vi "ContextHelp_PopUp.vi"() -> ()   [LabVIEW 2012]
uses:
  <resource>/Framework/Providers/Open_GDS/UML/ContextHelp/ContextHelp_EventType.ctl
  <resource>/Framework/Providers/Open_GDS/UML/ContextHelp/ContextHelp_ShowType.ctl
  <vilib>/event_ctls.llb/eventvkey.ctl
panel:
  in  "CallerRef":refnum<vi>
  in  "OccSync":refnum<k4>
  in  "Event":T1
  out "new picture":picture
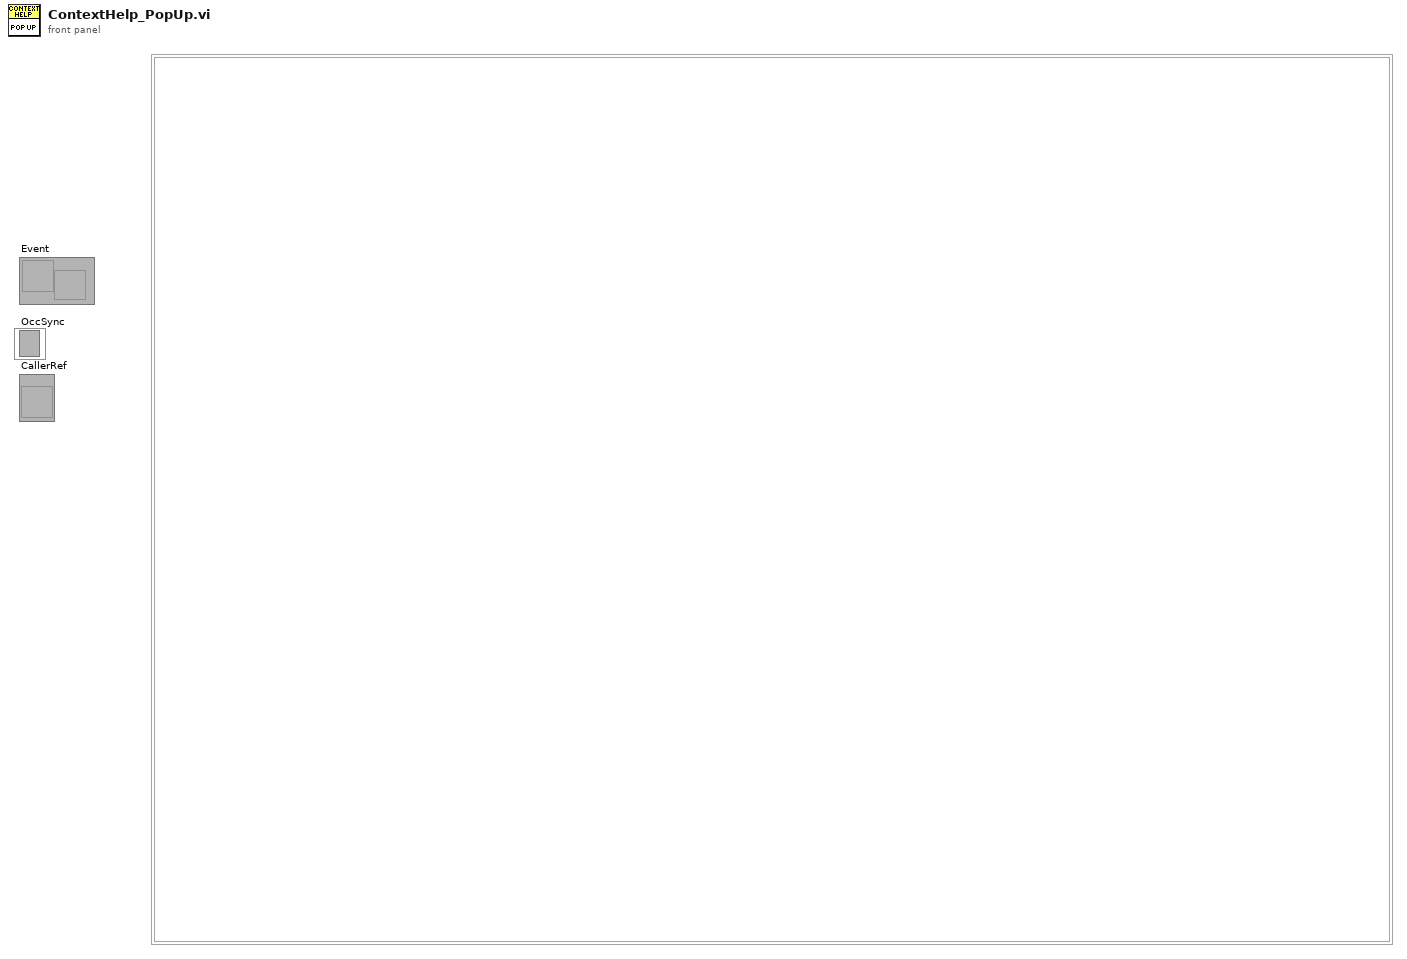
[diagram p1: front panel]
types:
  T1 = typedef "ContextHelp_EventType.ctl" = refnum<user-event>
  T2 = typedef "ContextHelp_ShowType.ctl" = cluster{"Header":string, "Picture":picture, "Text":string}
  T3 = cluster{"VIs":refnum<vi>[], "ViPathes":path[], "VI":i32, "Show":T2, "Win":cluster{"left":i16, "top":i16, "right":i16, "bottom":i16}, "LastViRef":refnum<vi>}
  T4 = enum32{"Custom", "Standard", "Using Panel", "Using SubVI", "Complete"}
  T5 = enum16{"SetPopUpEventTask", "GetStatus", "SetOpenState"}
  T6 = cluster{"left":i16, "top":i16, "right":i16, "bottom":i16}
  T7 = typedef "eventvkey.ctl" = enum16{"ASCII", "Enter", "Return", "Shift", "Ctrl", "Alt", "Cmd", "Opt", "Caps", "NumLock", "Clear", "Break", "Up", "Down", "Left", "Right", "Insert", "Delete", "Home", "End", "PageUp", "PageDown", "Escape", "Help", "Pause", "ScrollLock", "F1", "F2", "F3", "F4", "F5", "F6", "F7", "F8", "F9", "F10", "F11", "F12", "F13", "F14", "F15", "F16", "F17", "F18", "F19", "F20", "F21", "F22", "F23", "F24", "Play", "VolumeUp", "VolumeDown", "Mute", "Two Byte Char"}
  T8 = typedef "Librarian File Info Out.ctl" = cluster{"creation date":u32, "last mod date":u32, "type":string, "creator":string, "LV version":i32, "size":i32, "top level":bool}
  T9 = typedef "imagedata.ctl" = cluster{"image type":i32, "image depth":i32, "image":u8[], "mask":u8[], "colors":u32[], "Rectangle":cluster{"left":i16, "top":i16, "right":i16, "bottom":i16}}
  T10 = cluster{"Font Name:":string, "Size":i16, "Strikeout?":bool, "Italic?":bool, "Underline?":bool, "Outline?":bool, "Shadow?":bool, "Bold?":bool}
  T11 = enum16{"User-specified Font", "Application Font", "System Font", "Dialog Font"}
  T12 = typedef "LVRectTypeDef.ctl" = cluster{"Left":i16, "Top":i16, "Right":i16, "Bottom":i16}
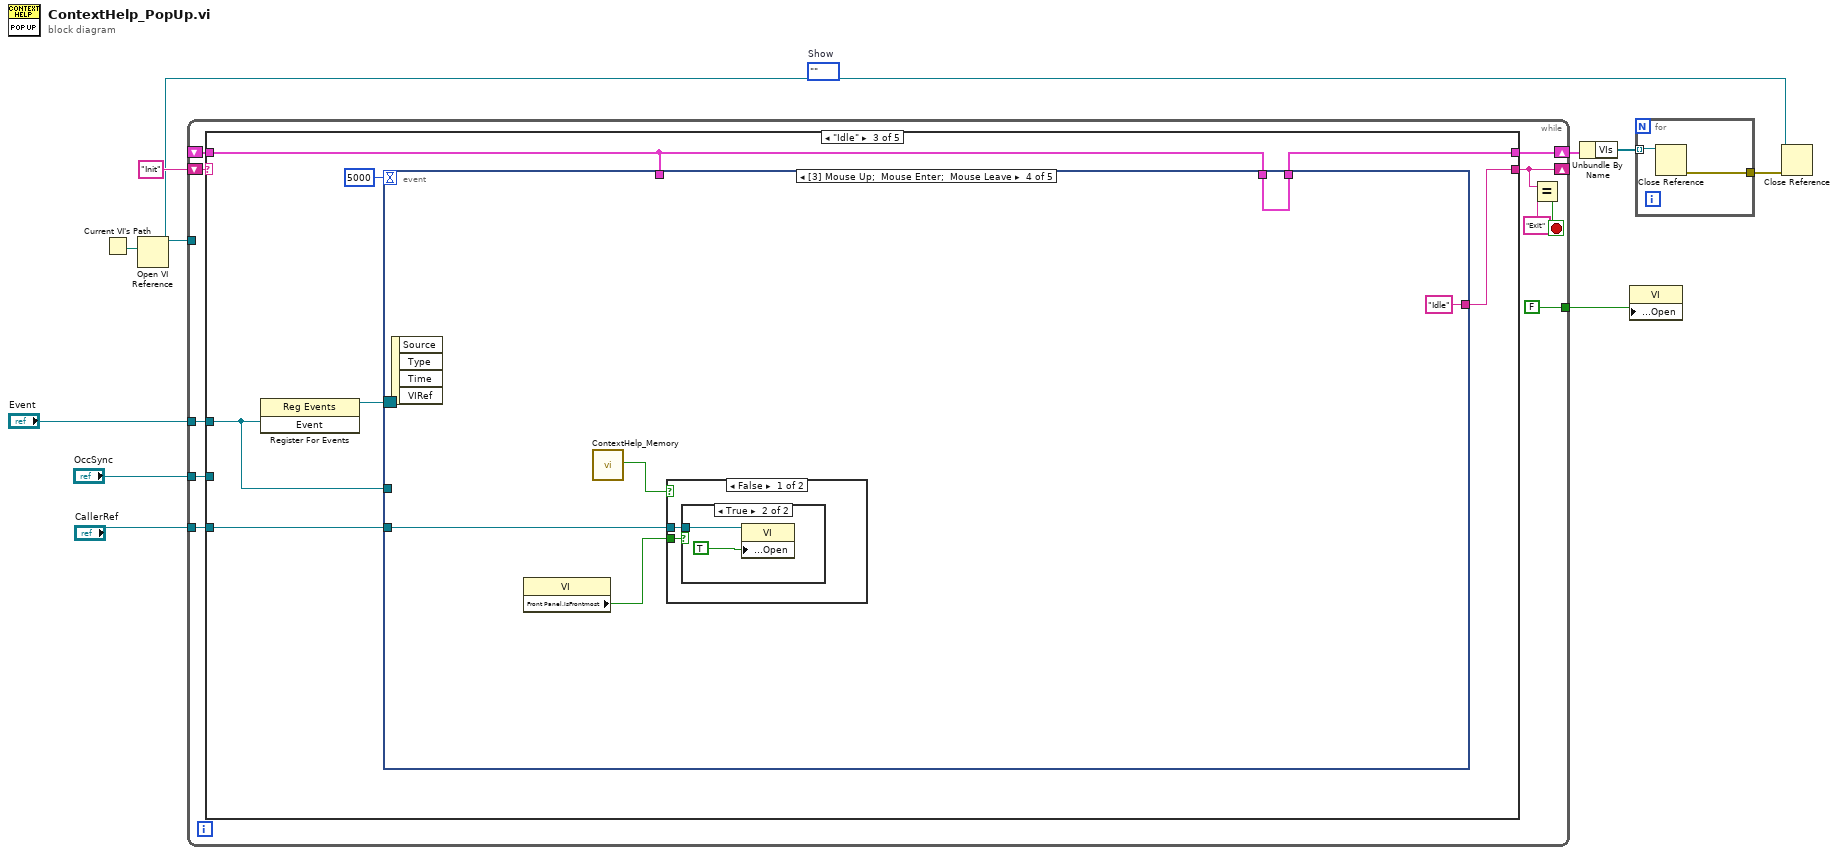
[diagram p0: block diagram]
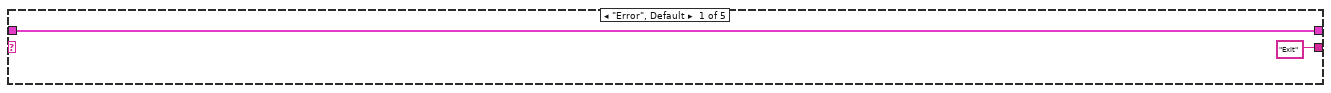
[diagram p2: hidden frame]
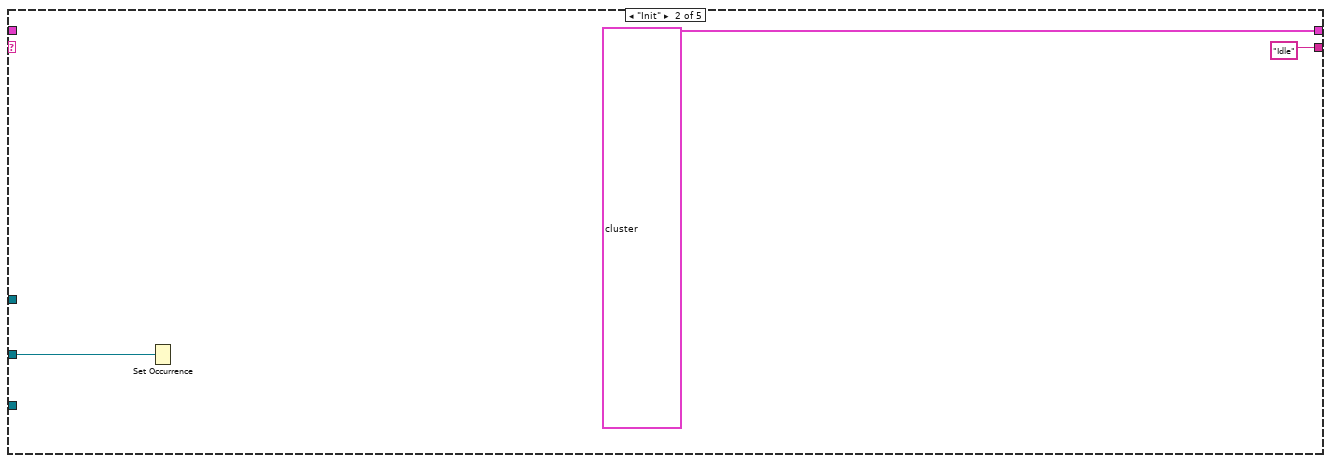
[diagram p3: hidden frame]
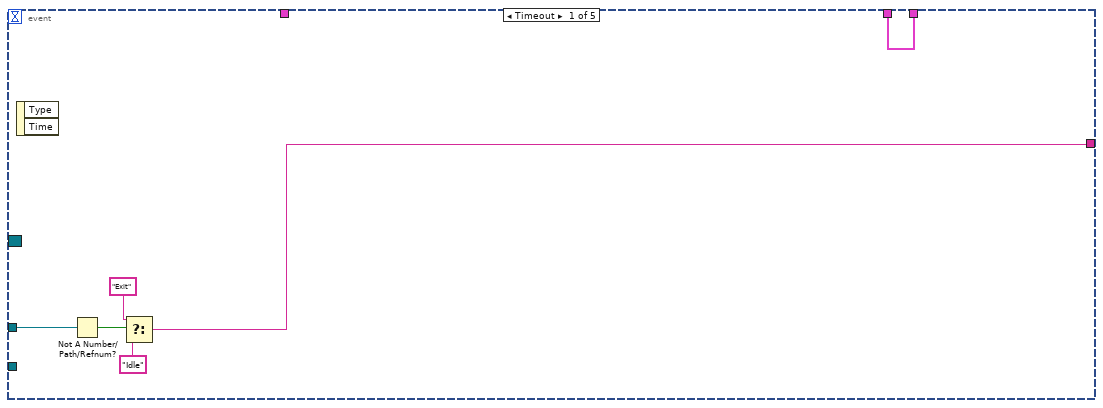
[diagram p4: hidden frame]
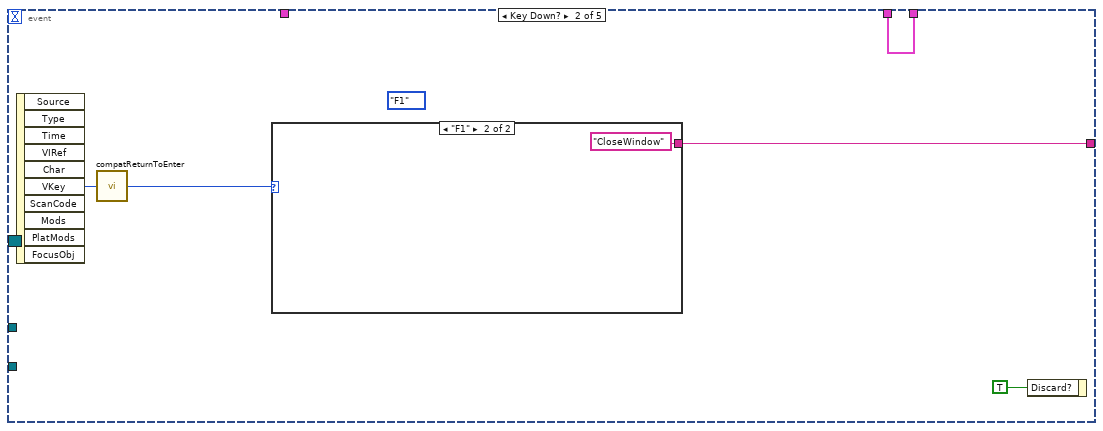
[diagram p5: hidden frame]
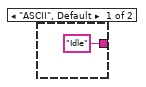
[diagram p6: hidden frame]
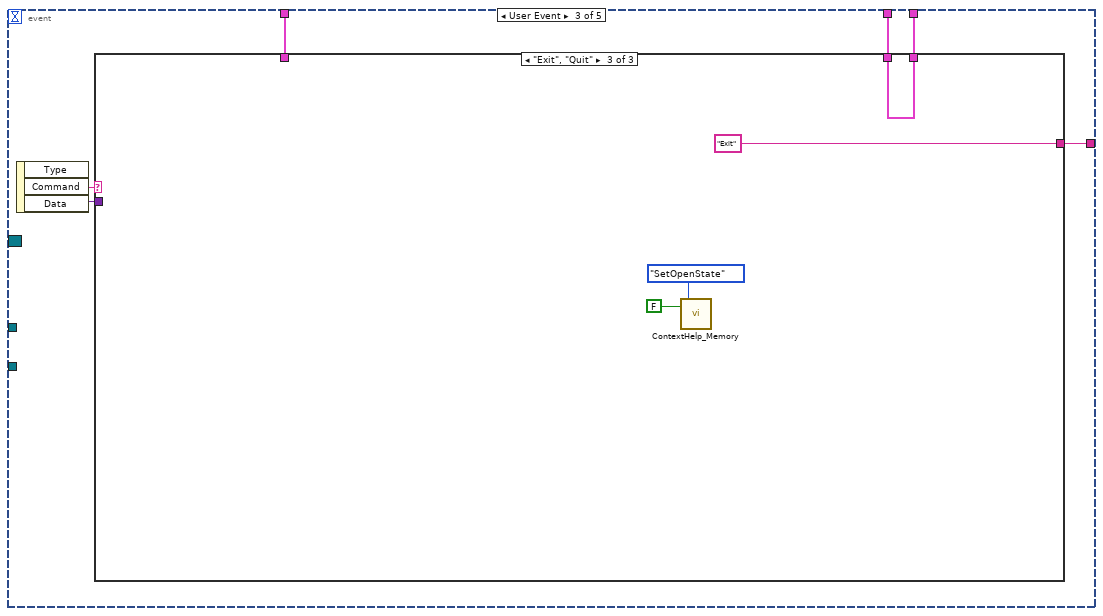
[diagram p7: hidden frame]
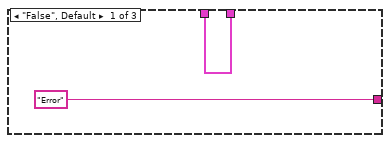
[diagram p8: hidden frame]
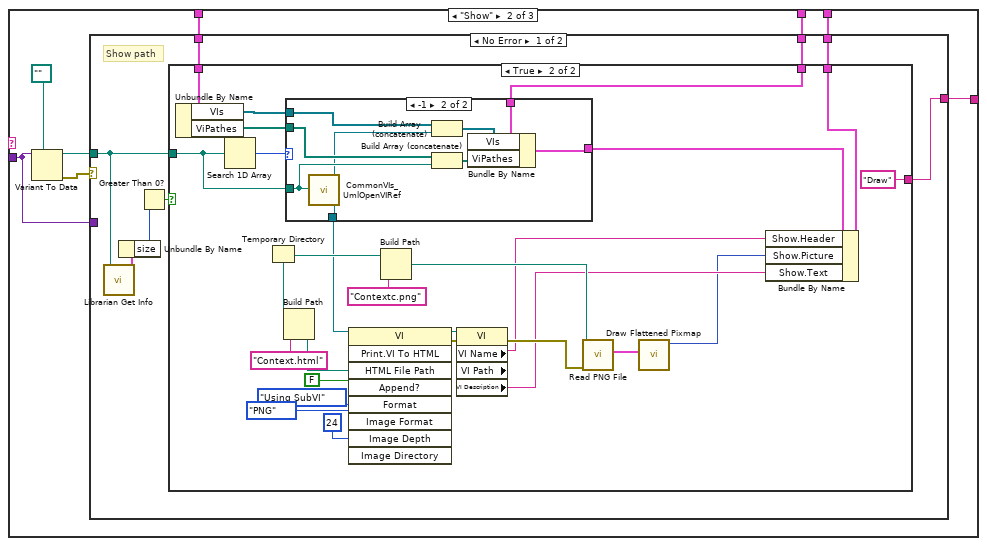
[diagram p9: hidden frame]
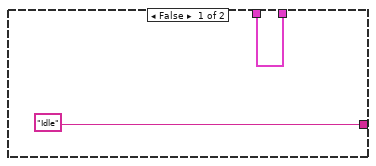
[diagram p10: hidden frame]
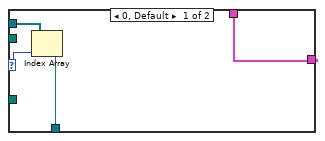
[diagram p11: hidden frame]
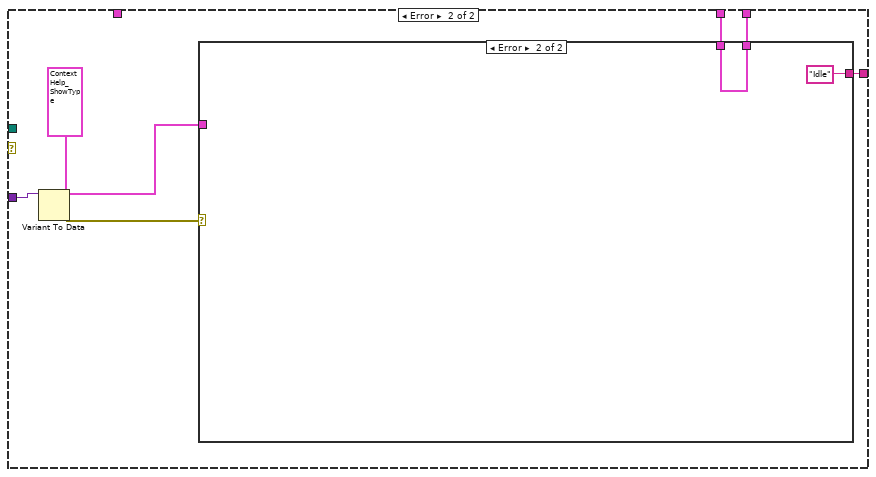
[diagram p12: hidden frame]
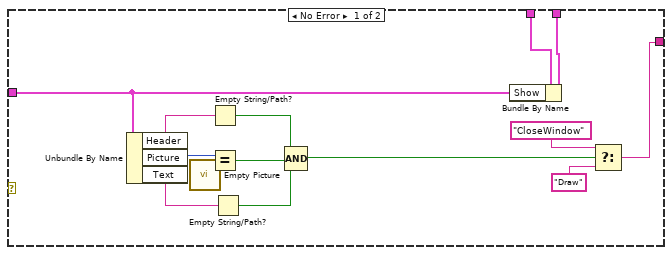
[diagram p13: hidden frame]
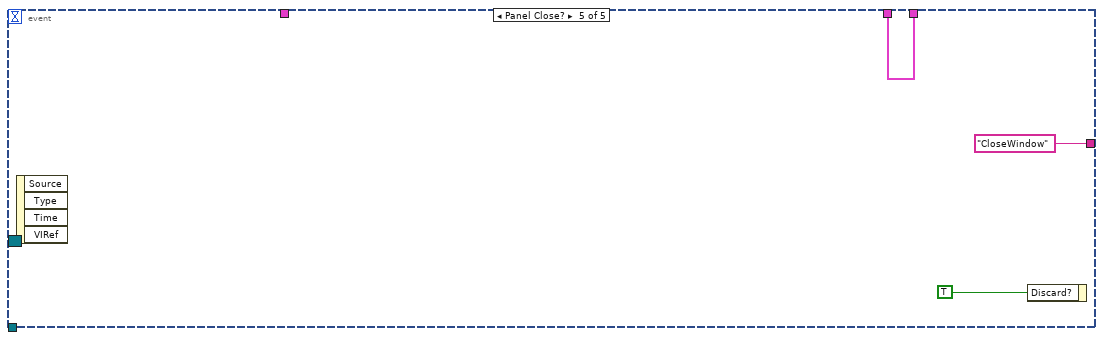
[diagram p16: hidden frame]
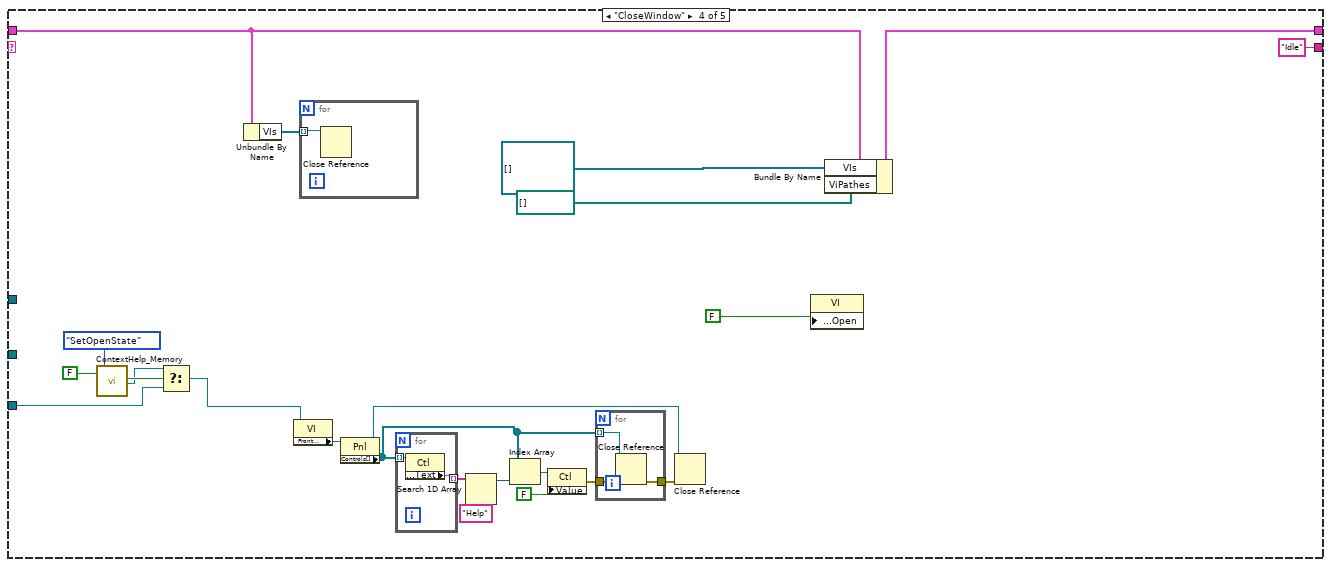
[diagram p17: hidden frame]
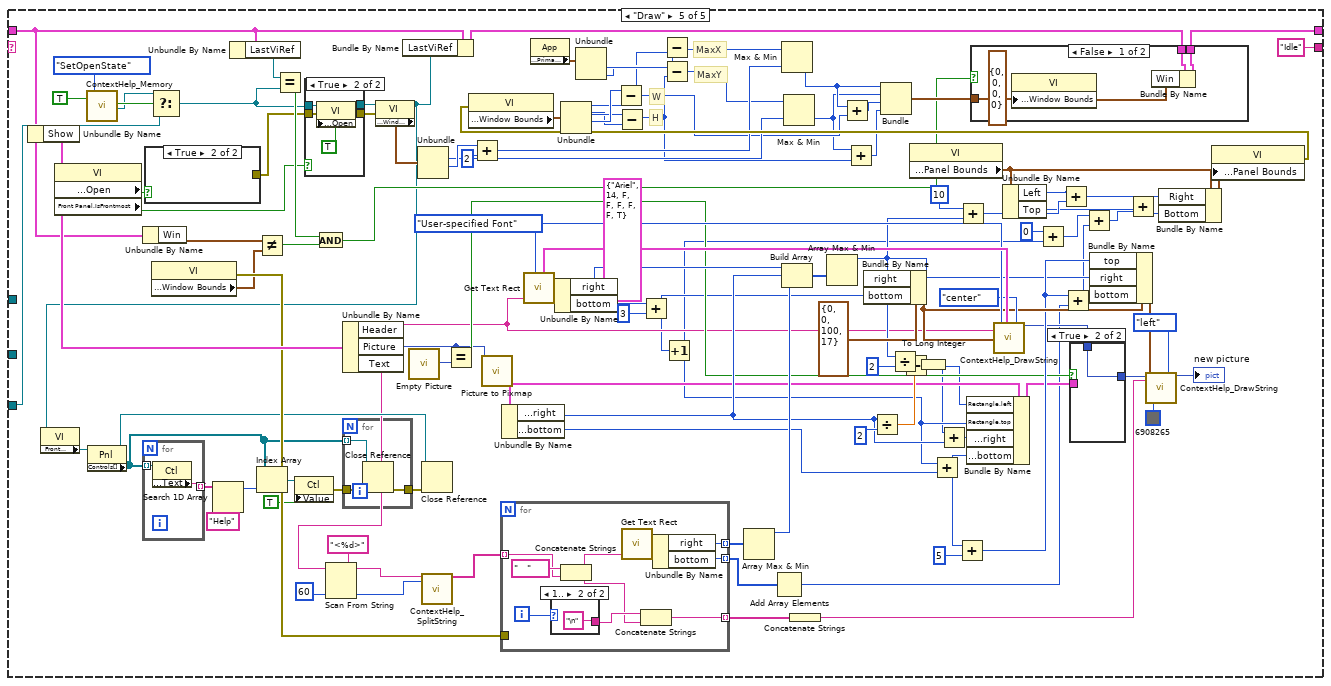
[diagram p18: hidden frame]
diagram:
  (unwired) enum16{"ClassDescription", ""}.""  # Show
  n1 = Current VI's Path() -> (path=w6:path)
  n2 = Open VI Reference(vi path=w6) -> (vi reference=w4:refnum<vi>)  [unwired: 2 in, 4 out]
  n3 = while {
    shift-right: [w19] -> _
    shift-left: "Init" -> [w20]
    shift-right: [w16] -> w8
    shift-left: _ -> [w15]
    tunnel: "Event" -> [w14]
    tunnel: w4 -> [_]
    tunnel: "OccSync" -> [w13]
    tunnel: [FALSE ("Front Panel Window:Open")] -> w2
    tunnel: "CallerRef" -> [w11]
    stop <- w17 stop-if-true
    n4 = case shown="\"Idle\"" w20 {
      tunnel: ["Exit" "Idle" w31 "Idle" "Idle"] -> w19
      tunnel: [w21 T3 {"VIs"=[], "ViPathes"=[], "VI"=0, "Show"={"Header"="", "Picture"=bytes[0], "Text"=""}, "Win"={"left"=0, "top"=0, "right"=0, "bottom"=0}, "LastViRef"=refnum} w30 w156 w207] -> w16
      tunnel: w15 -> [w21 _ w29 w157 w205]
      tunnel: w14 -> [_ _ w27 _ _]
      tunnel: w13 -> [_ w23 _ _ _]
      tunnel: w11 -> [_ _ w26 w150 w233]
      frame "Error", Default {
      }
      frame "Init" {
        n5 = Set Occurrence(w23) -> ()
      }
      frame "Idle" {
        n6 = register-events(w27) -> (reference out=w32:refnum<event-registration>)  [unwired: 2 in, 1 out]
        n7 = event shown="[3] Mouse Up;  Mouse Enter;  Mouse Leave" {
          selector: w32 -> [_ _ _ _ _]
          dyn-events: _ -> [_ _ _ _ _]
          timeout: 5000 -> [_ _ _ _ _]
          tunnel: [w34 w41 w50 "Idle" "CloseWindow"] -> w31
          tunnel: w29 -> [w38 w43 w49 w141 w146]
          tunnel: [w38 w43 w48 w141 w146] -> w30
          tunnel: w29 -> [_ _ w46 _ _]
          tunnel: w27 -> [w37 _ _ _ _]
          tunnel: w26 -> [_ _ _ w139 _]
          event Timeout {
            n8 = event-data() -> ()  [unwired: 3 out]
            n9 = Not A Number/Path/Refnum?(number/path/refnum=w37) -> (NaN/Path/Refnum?=w36:bool)
            n10 = Select(t="Exit", s=w36, f="Idle") -> (s? t:f=w34:string)
          }
          event Key Down? {
            (unwired) eventvkey."F1" ("VKey")
            n11 = event-data() -> ("VKey"=w39:T7)  [unwired: 10 out]
            n12 = call <vilib>:"compatReturnToEnter.vi"("VKey"=w39) -> ("VKey"=w42:T7)
            n13 = case shown="\"F1\"" w42 {
              tunnel: ["Idle" "CloseWindow"] -> w41
              frame "ASCII", Default {
              }
              frame "F1" {
              }
            }
            n14 = event-data("Discard?"=TRUE) -> ()  [unwired: 1 in, 1 out]
          }
          event User Event {
            n15 = event-data() -> ("Command"=w51:string, "Data"=w47:variant)  [unwired: 2 out]
            n16 = case shown="\"Exit\", \"Quit\"" w51 {
              tunnel: ["Error" w56 "Exit"] -> w50
              tunnel: w49 -> [w53 w59 w135]
              tunnel: [w53 w58 w135] -> w48
              tunnel: w47 -> [_ w54 _]
              tunnel: w46 -> [_ w60 _]
              frame "False", Default {
              }
              frame "Show" {
                n17 = Variant To Data(type=path "", Variant=w54) -> (data=w57:path, error out=w55:errorcluster)  [unwired: 1 in]
                n18 = case shown="No Error" w55 {
                  tunnel: w60 -> [w69 _]
                  tunnel: w59 -> [w68 w115]
                  tunnel: [w67 w114] -> w58
                  tunnel: w57 -> [w65 _]
                  tunnel: [w66 w111] -> w56
                  tunnel: w54 -> [_ w116]
                  frame No Error {
                    # "Show path"
                    n19 = call <vilib>:"Librarian Get Info.vi"("path"=w65) -> ("file information"=w64:T8)  [unwired: 1 in, 9 out]
                    n20 = Unbundle By Name(w64) -> ("size"=w63:i32)
                    n21 = Greater Than 0?(x=w63) -> (x > 0?=w62:bool)
                    n22 = case shown="True" w62 {
                      tunnel: w69 -> [_ w97]
                      tunnel: w68 -> [w71 w95]
                      tunnel: [w71 w90] -> w67
                      tunnel: w65 -> [_ w92]
                      tunnel: ["Idle" "Draw"] -> w66
                      frame False {
                      }
                      frame True {
                        n23 = Unbundle By Name(w97) -> ("VIs"=w94:refnum<vi>[], "ViPathes"=w93:path[])
                        n24 = Search 1D Array(1D array=w93, element=w92) -> (index of element=w96:i32)  [unwired: 1 out]
                        n25 = Temporary Directory() -> (w81:path)
                        n26 = Build Path(base path=w81, name or relative path="Context.html") -> (appended path=w79:path)
                        n27 = case shown="-1" w96 {
                          selector: w96 -> [w101 _]
                          tunnel: w92 -> [_ w103]
                          tunnel: w95 -> [w98 w109]
                          tunnel: w94 -> [w100 w108]
                          tunnel: w93 -> [_ w105]
                          tunnel: [w98 w104] -> w89
                          tunnel: [w99 w102] -> w76
                          frame 0, Default {
                            n28 = Index Array(array=w100, index=w101) -> (element=w99:refnum<vi>)
                          }
                          frame -1 {
                            n29 = call <resource>:"CommonVIs_UmlOpenVIRef.vi"("ViPath/ViName"=w103) -> ("vi reference"=w102:refnum<vi>)  [unwired: 3 in, 7 out]
                            n30 = Build Array (concatenate)(w108, w102) -> (w107:refnum<vi>[])
                            n31 = Build Array (concatenate)(w105, w103) -> (w106:path[])
                            n32 = Bundle By Name(cluster=w109, "VIs"=w107, "ViPathes"=w106) -> (w104:T3)
                          }
                        }
                        n33 = invoke class="VI" method="Print.VI To HTML"(reference=w76, "HTML File Path"=w79, "Append?"=FALSE, "Format"=T4."Using SubVI", "Image Format"=enum32{"PNG", "JPEG", "GIF"}."PNG", "Image Depth"=24) -> (reference out=w86:refnum<vi>, error out=w85:errorcluster)  [unwired: 3 in, 7 out]
                        n34 = Build Path(base path=w81, name or relative path="Contextc.png" ("HTML File Path")) -> (appended path=w78:path)
                        n35 = property class="VI" props=["VI Name", "VI Path", "VI Description"](reference=w86, error in=w85) -> (error out=w84:errorcluster, "VI Name"=w75:string, "VI Description"=w74:string)  [unwired: 2 out]
                        n36 = call <vilib>:"Read PNG File.vi"("error in (no error)"=w84, "path to PNG file"=w78) -> ("image data"=w73:T9)  [unwired: 9 out]
                        n37 = call <vilib>:"Draw Flattened Pixmap.vi"("image data"=w73) -> ("new picture"=w72:picture)  [unwired: 1 in, 7 out]
                        n38 = Bundle By Name(cluster=w89, "Show.Header"=w75, "Show.Picture"=w72, "Show.Text"=w74) -> (w90:T3)
                      }
                    }
                  }
                  frame Error {
                    n39 = Variant To Data(type=T2 {"Header"="", "Picture"=bytes[0], "Text"=""} ("output cluster"), Variant=w116) -> (data=w113:T2, error out=w112:errorcluster)  [unwired: 1 in]
                    n40 = case shown="Error" w112 {
                      tunnel: w115 -> [w130 w131]
                      tunnel: [w129 w131] -> w114
                      tunnel: w113 -> [w128 _]
                      tunnel: [w119 "Idle"] -> w111
                      frame No Error {
                        n41 = Unbundle By Name(w128) -> ("Header"=w124:string, "Picture"=w127:picture, "Text"=w125:string)
                        n42 = call "Empty Picture"() -> ("empty picture"=w126:picture)
                        n43 = Empty String/Path?(string/path=w124) -> (empty?=w123:bool)
                        n44 = Equal?(x=w127, y=w126) -> (x = y?=w122:bool)
                        n45 = Empty String/Path?(string/path=w125) -> (empty?=w121:bool)
                        n46 = Compound Arithmetic op=AND(w123, w122, w121) -> (w117:bool)
                        n47 = Bundle By Name(cluster=w130, "Show"=w128) -> (w129:T3)
                        n48 = Select(t="CloseWindow", s=w117, f="Draw") -> (s? t:f=w119:string)
                      }
                      frame Error {
                      }
                    }
                  }
                }
              }
              frame "Exit", "Quit" {
                n49 = call <resource>:"ContextHelp_Memory.vi"("State"=FALSE ("OpenState"), "Actio(GetStatus)n"=T5."SetOpenState") -> ()  [unwired: 2 in, 16 out]
              }
            }
          }
          event Mouse Up; Mouse Enter; Mouse Leave {
            n50 = event-data() -> ()  [unwired: 5 out]
            n51 = property class="VI"() -> ("Front Panel.IsFrontmost"=w137:bool)  [unwired: 2 in, 2 out]
            n52 = call <resource>:"ContextHelp_Memory.vi"() -> ("DialogCaller"=w138:bool)  [unwired: 4 in, 15 out]
            n53 = case shown="False" w138 {
              tunnel: w139 -> [w143 _]
              tunnel: w137 -> [w142 _]
              frame False {
                n54 = case shown="True" w142 {
                  tunnel: w143 -> [_ w145]
                  frame False {
                  }
                  frame True {
                    n55 = property class="VI"(reference=w145, "Front Panel Window:Open"=TRUE ("Front Panel Window:Is Frontmost")) -> ()  [unwired: 1 in, 2 out]
                  }
                }
              }
              frame True {
              }
            }
          }
          event Panel Close? {
            n56 = event-data() -> ()  [unwired: 5 out]
            n57 = event-data("Discard?"=TRUE) -> ()  [unwired: 1 in, 1 out]
          }
        }
      }
      frame "CloseWindow" {
        n58 = call <resource>:"ContextHelp_Memory.vi"("State"=FALSE ("OpenState"), "Actio(GetStatus)n"=T5."SetOpenState") -> ("DialogCaller"=w152:bool, "DialogRef"=w151:refnum<vi>)  [unwired: 2 in, 14 out]
        n59 = Select(t=w151, s=w152, f=w150) -> (s? t:f=w149:refnum<vi>)
        n60 = Unbundle By Name(w157) -> ("VIs"=w170:refnum<vi>[])
        n61 = property class="VI"(reference=w149) -> ("Front Panel"=w167:refnum<vi>)  [unwired: 1 in, 2 out]
        n62 = for {
          tunnel: w170 -> [w177] mode=indexing
          n63 = Close Reference(reference=w177) -> ()  [unwired: 1 in, 1 out]
        }
        n64 = property class="Pnl"(reference=w167) -> (reference out=w158:refnum<vi>, "Controls[]"=w160:refnum<vi>[])  [unwired: 1 in, 1 out]
        n65 = for {
          tunnel: w160 -> [w176] mode=indexing
          tunnel: [w175] -> w166 mode=indexing
          n66 = property class="Ctl"(reference=w176) -> ("Label.Text"=w175:string)  [unwired: 1 in, 2 out]
        }
        n67 = Search 1D Array(1D array=w166, element="Help") -> (index of element=w164:i32)  [unwired: 1 out]
        n68 = Index Array(array=w160, index=w164) -> (element=w163:refnum<vi>)
        n69 = property class="Ctl"(reference=w163, "Value"=FALSE ("Discard?")) -> (error out=w161:errorcluster)  [unwired: 1 in, 1 out]
        n70 = for {
          tunnel: w161 -> [w174]
          tunnel: w160 -> [w173] mode=indexing
          tunnel: [w172] -> w159
          n71 = Close Reference(reference=w173, error in (no error)=w174) -> (error out=w172:errorcluster)
        }
        n72 = Close Reference(reference=w158, error in (no error)=w159) -> ()  [unwired: 1 out]
        n73 = property class="VI"("Front Panel Window:Open"=FALSE) -> ()  [unwired: 2 in, 2 out]
        n74 = Bundle By Name(cluster=w157, "VIs"=refnum<vi>[] [], "ViPathes"=path[] []) -> (w156:T3)
      }
      frame "Draw" {
        w290 = T10 {"Font Name:"="Ariel", "Size"=14, "Strikeout?"=FALSE, "Italic?"=FALSE, "Underline?"=FALSE, "Outline?"=FALSE, "Shadow?"=FALSE, "Bold?"=TRUE} ("[user-specified font]")
        w289 = T11."User-specified Font" ("desired font(Application)")
        # "MaxX"
        # "MaxY"
        # "H"
        # "W"
        n75 = Unbundle By Name(w205) -> ("Show"=w253:T2)
        n76 = property class="VI"() -> ("Front Panel Window:Open"=w238:bool, "Front Panel.IsFrontmost"=w178:bool)  [unwired: 2 in, 2 out]
        n77 = call <resource>:"ContextHelp_Memory.vi"("State"=TRUE ("OpenState"), "Actio(GetStatus)n"=T5."SetOpenState") -> ("DialogCaller"=w234:bool, "DialogRef"=w232:refnum<vi>)  [unwired: 2 in, 14 out]
        n78 = Unbundle By Name(w205) -> ("Win"=w203:T6)
        n79 = case shown="True" w238 {
          tunnel: [w312 _] -> w181
          frame False {
            n80 = property class="VI"("Front Panel Window:Open"=TRUE) -> (error out=w312:errorcluster)  [unwired: 2 in, 1 out]
          }
          frame True {
          }
        }
        n81 = Select(t=w232, s=w234, f=w233) -> (s? t:f=w182:refnum<vi>)
        n82 = property class="VI"() -> (error out=w208:errorcluster, "Front Panel Window:Window Bounds"=w204:T12)  [unwired: 2 in, 1 out]
        n83 = Unbundle By Name(w205) -> ("LastViRef"=w202:refnum<vi>)
        n84 = Not Equal?(x=w203, y=w204) -> (x != y?=w201:bool)
        n85 = Equal?(x=w202, y=w182) -> (x = y?=w183:bool)
        n86 = case shown="True" w178 {
          tunnel: w182 -> [w297 w302]
          tunnel: w181 -> [w296 w301]
          tunnel: [w297 w300] -> w180
          tunnel: [w296 w299] -> w179
          frame False {
          }
          frame True {
            n87 = property class="VI"(reference=w302, error in=w301, "Front Panel Window:Open"=TRUE) -> (reference out=w300:refnum<vi>, error out=w299:errorcluster)
          }
        }
        n88 = And(x=w183, y=w201) -> (x .and. y?=w200:bool)
        n89 = Unbundle By Name(w253) -> ("Header"=w248:string, "Picture"=w250:picture, "Text"=w184:string)
        n90 = Scan From String(format string="<%d>" ("regular expression"), input string=w184, default 1=60 ("Max string length")) -> (remaining string=w185:string, output 1=w186:i32)  [unwired: 2 in, 2 out]
        n91 = property class="VI"(reference=w180, error in=w179) -> (reference out=w189:refnum<vi>, "Front Panel Window:Window Bounds"=w222:T12)  [unwired: 1 out]
        n92 = property class="VI"(reference=w189) -> ("Front Panel"=w199:refnum<vi>)  [unwired: 1 in, 2 out]
        n93 = property class="Pnl"(reference=w199) -> (reference out=w190:refnum<vi>, "Controls[]"=w192:refnum<vi>[])  [unwired: 1 in, 1 out]
        n94 = for {
          tunnel: w192 -> [w307] mode=indexing
          tunnel: [w306] -> w198 mode=indexing
          n95 = property class="Ctl"(reference=w307) -> ("Label.Text"=w306:string)  [unwired: 1 in, 2 out]
        }
        n96 = Search 1D Array(1D array=w198, element="Help") -> (index of element=w196:i32)  [unwired: 1 out]
        n97 = Index Array(array=w192, index=w196) -> (element=w195:refnum<vi>)
        n98 = property class="Ctl"(reference=w195, "Value"=TRUE ("Discard?")) -> (error out=w193:errorcluster)  [unwired: 1 in, 1 out]
        n99 = for {
          tunnel: w193 -> [w305]
          tunnel: w192 -> [w304] mode=indexing
          tunnel: [w303] -> w191
          n100 = Close Reference(reference=w304, error in (no error)=w305) -> (error out=w303:errorcluster)
        }
        n101 = Bundle By Name(cluster=w205, "LastViRef"=w189) -> (w206:T3)
        n102 = call "Empty Picture"() -> ("empty picture"=w252:picture)
        n103 = Unbundle(w222) -> ("Top"=w215:i16, "Right"=w221:i16)  [unwired: 2 out]
        n104 = Close Reference(reference=w190, error in (no error)=w191) -> ()  [unwired: 1 out]
        n105 = call <resource>:"ContextHelp_SplitString.vi"("string"=w185, "Max string length"=w186) -> ("Array"=w256:string[])  [unwired: 17 out]
        n106 = Equal?(x=w250, y=w252) -> (x = y?=w251:bool)
        n107 = Add(x=w221, y=i16 2) -> (x+y=w217:i16)
        n108 = call <vilib>:"Picture to Pixmap.vi"("picture"=w250) -> ("image data"=w249:T9)  [unwired: 3 in, 7 out]
        n109 = for {
          tunnel: w256 -> [w322] mode=indexing
          tunnel: [w325] -> w294 mode=indexing
          tunnel: [w324] -> w240 mode=indexing
          tunnel: [w321] -> w255 mode=indexing
          tunnel: w208 -> [_]
          i -> [w320]
          n110 = case shown="1.." w320 {
            tunnel: ["" "\n"] -> w319
            frame 0, Default {
            }
            frame 1.. {
            }
          }
          n111 = Concatenate Strings("   " ("replace string (\"\")"), w322) -> (w318:string)
          n112 = call <vilib>:"Get Text Rect.vi"("text"=w318) -> ("rect"=w326:T6)  [unwired: 5 in, 3 out]
          n113 = Concatenate Strings(w319, w318) -> (w321:string)
          n114 = Unbundle By Name(w326) -> ("right"=w325:i16, "bottom"=w324:i16)
        }
        n115 = Unbundle By Name(w249) -> ("Rectangle.right"=w279:i16, "Rectangle.bottom"=w280:i16)
        n116 = call <vilib>:"Get Text Rect.vi"("desired font(Application)"=w289, "text"=w248, "[user-specified font]"=w290) -> ("rect"=w295:T6)  [unwired: 3 in, 3 out]
        n117 = property class="App"() -> ("Display:Primary Workspace"=w225:T12)  [unwired: 2 in, 2 out]
        n118 = Unbundle By Name(w295) -> ("right"=w293:i16, "bottom"=w247:i16)
        n119 = Unbundle(w225) -> ("Right"=w224:i16, "Bottom"=w223:i16)  [unwired: 2 out]
        n120 = Add(x=w247, y=i16 3) -> (x+y=w245:i16)
        n121 = Increment(x=w245) -> (x+1=w241:i16)
        n122 = Array Max & Min(array=w294) -> (max value=w292:i16)  [unwired: 3 out]
        n123 = Add Array Elements(numeric array=w240) -> (sum=w239:i16)
        n124 = Build Array(w293, w279, w292) -> (w291:i16[])
        n125 = Concatenate Strings(w255) -> (w254:string)
        n126 = Array Max & Min(array=w291) -> (max value=w265:i16)  [unwired: 3 out]
        n127 = Bundle By Name(cluster=T6 {"left"=0, "top"=0, "right"=100, "bottom"=17} ("rect"), "right"=w265, "bottom"=w245) -> (w274:T6)
        n128 = Divide(x=w279, y=i16 2) -> (x/y=w283:dbl)
        n129 = Divide(x=w265, y=i16 2) -> (x/y=w285:dbl)
        n130 = Subtract(x=w285, y=w283) -> (x-y=w282:dbl)
        n131 = property class="VI"() -> ("Front Panel Window:Panel Bounds"=w267:T12)  [unwired: 2 in, 2 out]
        n132 = To Long Integer(number=w282) -> (32bit integer=w235:i32)
        n133 = Add(x=w241, y=w280) -> (x+y=w273:i16)
        n134 = Add(x=w235, y=w279) -> (x+y=w281:i32)
        n135 = Add(x=w273, y=i16 5) -> (x+y=w271:i16)
        n136 = Add(x=i16 10, y=w265) -> (x+y=w264:i16)
        n137 = Bundle By Name(cluster=w249, "Rectangle.left"=w235, "Rectangle.top"=w241, "Rectangle.right"=w281, "Rectangle.bottom"=w273) -> (w269:T9)
        n138 = call <resource>:"ContextHelp_DrawString.vi"("Text"=w248, "rect"=w274, "desired font(Application)"=w289, "[user-specified font]"=w290, "Justify(center)"=enum16{"left", "center", "right"}."center") -> ("PictureOut"=w257:picture)  [unwired: 8 in, 6 out]
        n139 = Unbundle By Name(w267) -> ("Left"=w266:i16, "Top"=w260:i16)
        n140 = Add(x=i16 0, y=w241) -> (x+y=w243:i16)
        n141 = Add(x=w266, y=w264) -> (x+y=w262:i16)
        n142 = Add(x=w271, y=w239) -> (x+y=w263:i16)
        n143 = case shown="True" w251 {
          tunnel: [w316 w317] -> w278
          tunnel: w269 -> [w315 _]
          tunnel: w257 -> [w314 w317]
          frame False {
            n144 = call <vilib>:"Draw Flattened Pixmap.vi"("image data"=w315, "picture"=w314) -> ("new picture"=w316:picture)  [unwired: 7 out]
          }
          frame True {
          }
        }
        n145 = Add(x=w243, y=w263) -> (x+y=w259:i16)
        n146 = Bundle By Name(cluster=w274, "top"=w271, "right"=w265, "bottom"=w263) -> (w270:T6)
        n147 = Add(x=w260, y=w259) -> (x+y=w258:i16)
        n148 = call <resource>:"ContextHelp_DrawString.vi"("PictureIn"=w278, "Text"=w254, "rect"=w270, "text color(black)"=u32 6908265, "Justify(center)"=enum16{"left", "center", "right"}."left") -> ("PictureOut"=→"new picture":picture)  [unwired: 8 in, 6 out]
        n149 = Bundle By Name(cluster=w267, "Right"=w262, "Bottom"=w258) -> (w268:T12)
        n150 = property class="VI"("Front Panel Window:Panel Bounds"=w268) -> (error out=w231:errorcluster)  [unwired: 2 in, 1 out]
        n151 = property class="VI"(error in=w231) -> ("Front Panel Window:Window Bounds"=w230:T12)  [unwired: 1 in, 2 out]
        n152 = Unbundle(w230) -> ("Left"=w228:i16, "Top"=w226:i16, "Right"=w229:i16, "Bottom"=w227:i16)
        n153 = Subtract(x=w229, y=w228) -> (x-y=w212:i16)
        n154 = Subtract(x=w227, y=w226) -> (x-y=w209:i16)
        n155 = Subtract(x=w224, y=w212) -> (x-y=w218:i16)
        n156 = Subtract(x=w223, y=w209) -> (x-y=w216:i16)
        n157 = Max & Min(x=w218, y=w217) -> (min(x,y)=w214:i16)  [unwired: 1 out]
        n158 = Max & Min(x=w216, y=w215) -> (min(x,y)=w211:i16)  [unwired: 1 out]
        n159 = Add(x=w214, y=w212) -> (x+y=w213:i16)
        n160 = Add(x=w211, y=w209) -> (x+y=w210:i16)
        n161 = Bundle(w214, w211, w213, w210) -> (w219:cluster{i16, i16, i16, i16})  [unwired: 1 out]
        n162 = case shown="False" w200 {
          tunnel: w219 -> [w308 _]
          tunnel: w206 -> [w310 w311]
          tunnel: [w309 w311] -> w207
          frame False {
            (unwired) T6 {"left"=0, "top"=0, "right"=0, "bottom"=0} ("Front Panel Window:Window Bounds")
            n163 = property class="VI"("Front Panel Window:Window Bounds"=w308) -> ()  [unwired: 2 in, 2 out]
            n164 = Bundle By Name(cluster=w310, "Win"=w308) -> (w309:T3)
          }
          frame True {
          }
        }
      }
    }
    n165 = Equal?(x=w19, y="Exit") -> (x = y?=w17:bool)
  }
  n166 = Unbundle By Name(w8) -> ("VIs"=w7:refnum<vi>[])
  n167 = property class="VI"("Front Panel Window:Open"=w2) -> ()  [unwired: 2 in, 2 out]
  n168 = for {
    tunnel: w7 -> [w330] mode=indexing
    tunnel: [w329] -> w5
    n169 = Close Reference(reference=w330) -> (error out=w329:errorcluster)  [unwired: 1 in]
  }
  n170 = Close Reference(reference=w4, error in (no error)=w5) -> ()  [unwired: 1 out]
